vi "barebones control panel.vi"() -> ()   [LabVIEW 2012]
uses:
  JY-SPEX-TRIAX/controls.llb/Slits.ctl
  JY-SPEX-TRIAX/controls.llb/Turret Position (TRIAX).ctl
  Global/GPIB Numbers.vi
  JY-SPEX-TRIAX/JY-SPEX-TRIAX.lvlib
panel:
  out "wavelength at":dbl[unit]
  in  "Move to Wavelength":dbl[unit]
  in  "Read Wavelength":bool
  in  "Set Wavelength":bool
  in  "Read Grating":bool=TRUE
  out "Blaze Wavelength":dbl[unit]
  out "Groove Density":dbl[unit]
  in  "Set Grating":bool=TRUE
  in  "Grating position":T1
  in  "Set Mirror":bool=TRUE
  in  "position":enum16{"side (lateral)", "front (axial)"}(ring)
  in  "mirror":enum16{"entrance", "exit"}(ring)=enum."exit"
  in  "Read Slit":bool=TRUE
  out "Current Slit Position":dbl[unit]
  in  "Set Slit":bool=TRUE
  in  "Slit Entrance":T2
  in  "Desired Slit Position":dbl[unit]
  out "VISA out":refnum<visa-resource-name>
  out "error out":errorcluster
  in  "error in (no error)":errorcluster
  in  "Initialize":bool
  in  "stop":bool
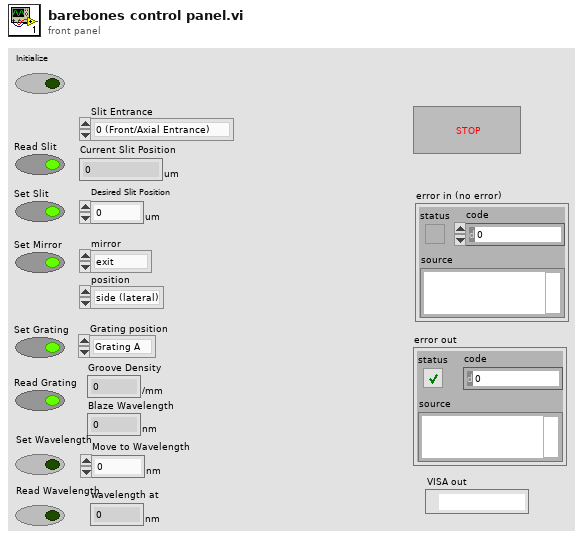
[diagram p1: front panel]
types:
  T1 = typedef "JY-SPEX-TRIAX.lvlib/Turret Position (TRIAX).ctl" = enum16{"Grating A", "Grating B", "Grating C"}
  T2 = typedef "JY-SPEX-TRIAX.lvlib/Slits.ctl" = enum16{"0 (Front/Axial Entrance)", "1 (Side/Lateral Entrance)", "2 (Front/Axial Exit)", "3 (Side/Lateral Exit)"}
  T3 = typedef "GPIB Type Def.ctl" = cluster{"Name":string, "bus":dbl, "GPIB":dbl, "GPIB as string":string, "byte":i32, "VISA Resource Name":refnum<visa-resource-name>}
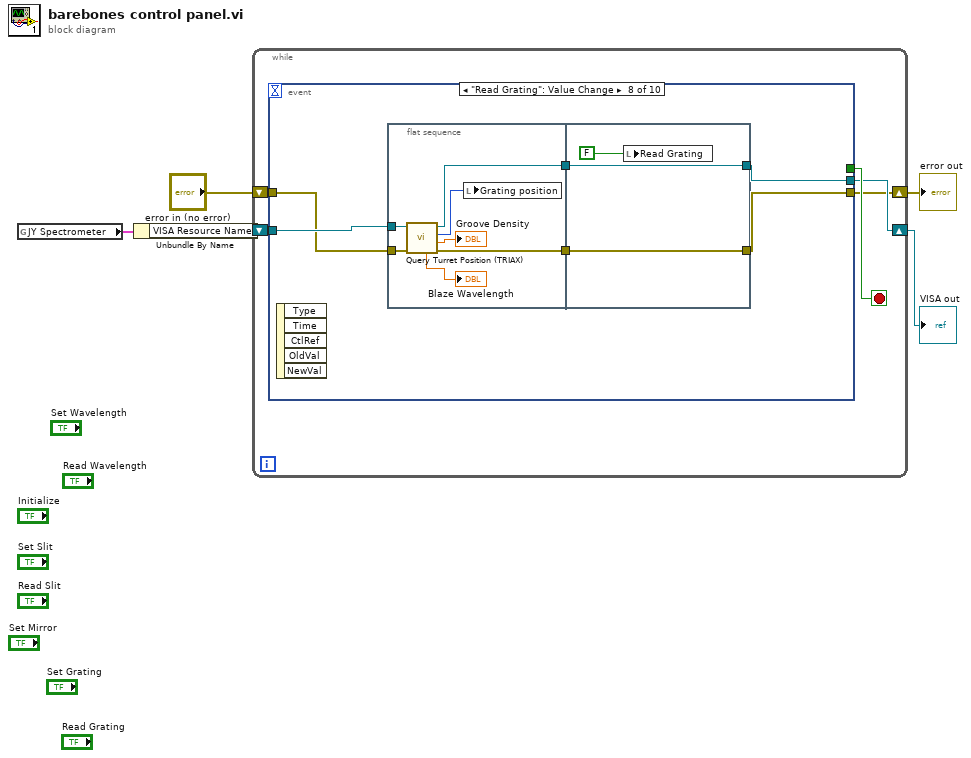
[diagram p0: block diagram]
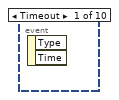
[diagram p2: hidden frame]
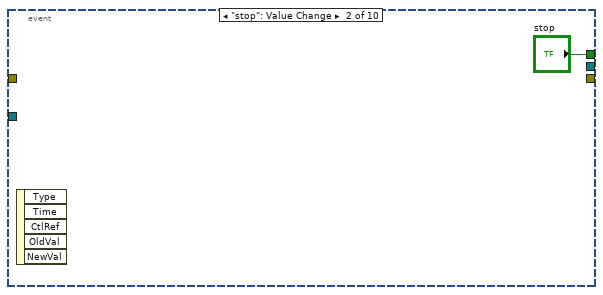
[diagram p3: hidden frame]
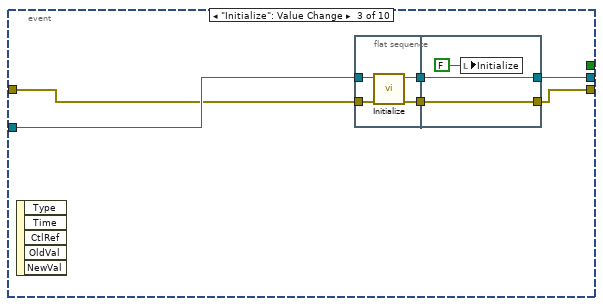
[diagram p4: hidden frame]
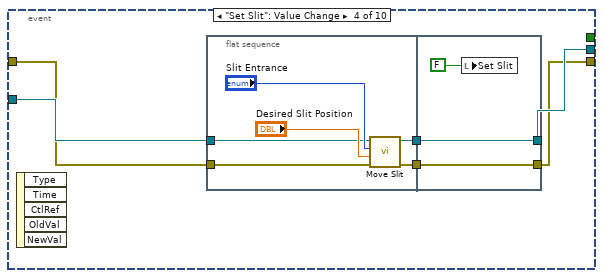
[diagram p5: hidden frame]
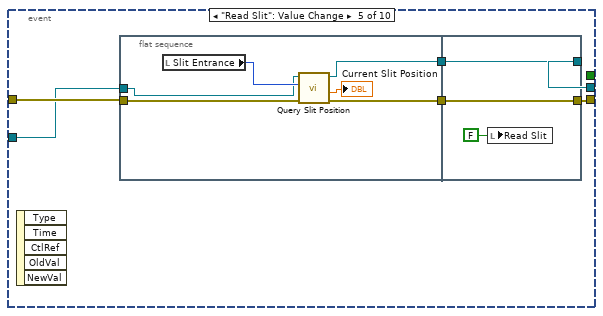
[diagram p6: hidden frame]
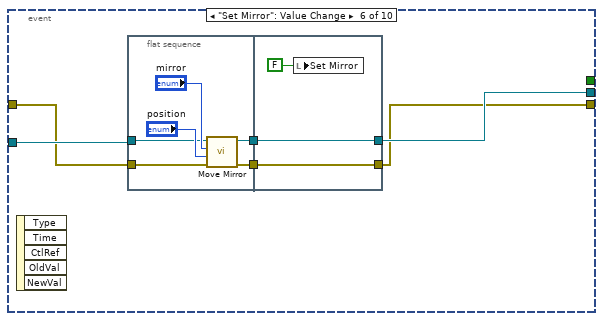
[diagram p7: hidden frame]
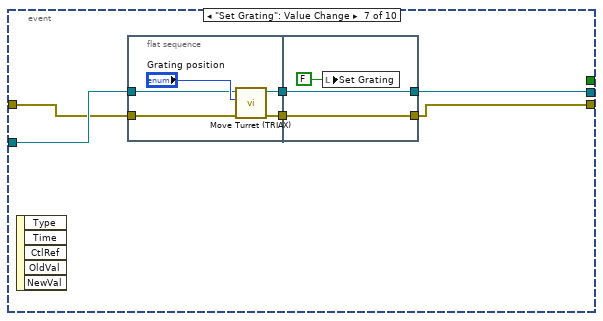
[diagram p8: hidden frame]
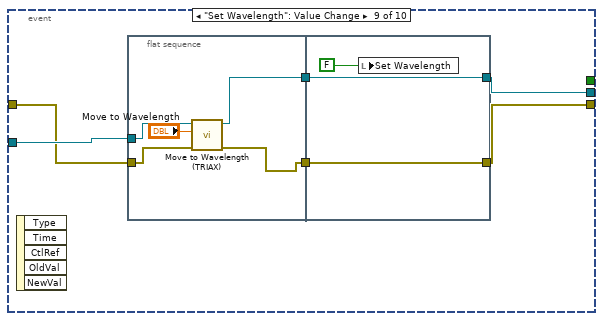
[diagram p9: hidden frame]
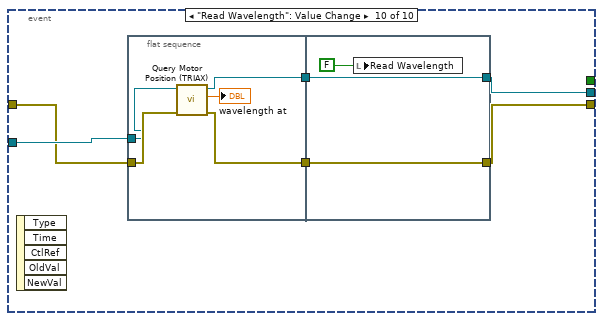
[diagram p10: hidden frame]
diagram:
  n1 = global read "GPIB Numbers.vi" "JY Spectrometer"() -> (w5:T3)
  n2 = Unbundle By Name(w5) -> ("VISA Resource Name"=w4:refnum<visa-resource-name>)
  n3 = while {
    shift-right: [w8] -> w1
    shift-left: w4 -> [w9]
    shift-right: [w6] -> w2
    shift-left: "error in (no error)" -> [w7]
    stop <- w10 stop-if-true
    n4 = event shown="[7] \"Read Grating\": Value Change" {
      selector: _ -> [_ _ _ _ _ _ _ _ _ _]
      dyn-events: _ -> [_ _ _ _ _ _ _ _ _ _]
      timeout: _ -> [_ _ _ _ _ _ _ _ _ _]
      tunnel: [_ "stop" _ _ _ _ _ _ _ _] -> w10
      tunnel: w9 -> [_ _ w17 w30 w42 w60 w75 w89 w105 w119]
      tunnel: w7 -> [_ _ w16 w27 w45 w59 w74 w88 w104 w118]
      tunnel: [_ _ w15 w29 w40 w57 w73 w87 w103 w117] -> w8
      tunnel: [_ _ w13 w26 w43 w55 w72 w86 w102 w116] -> w6
      event Timeout {
        n5 = event-data() -> ()  [unwired: 1 in, 2 out]
      }
      event "stop": Value Change {
        n6 = event-data() -> ()  [unwired: 1 in, 5 out]
      }
      event "Initialize": Value Change {
        n7 = event-data() -> ()  [unwired: 1 in, 5 out]
        n8 = flat-sequence {
          tunnel: w17 -> [w21]
          tunnel: w16 -> [w20]
          tunnel: [w19] -> w14
          tunnel: [w18] -> w12
          tunnel: [w23] -> w15
          tunnel: w14 -> [w23]
          tunnel: [w22] -> w13
          tunnel: w12 -> [w22]
          frame #0 {
            n9 = call "Initialize.vi"("error in (no error)"=w20, "VISA resource name"=w21) -> ("error out"=w18:errorcluster, "VISA resource name out"=w19:refnum<visa-resource-name>)  [unwired: 8 in]
          }
          frame #1 {
            n10 = local write "Initialize"(FALSE) -> ()
          }
        }
      }
      event "Set Slit": Value Change {
        n11 = event-data() -> ()  [unwired: 1 in, 5 out]
        n12 = flat-sequence {
          tunnel: w30 -> [w34]
          tunnel: [w33] -> w28
          tunnel: w27 -> [w32]
          tunnel: [w31] -> w25
          tunnel: [w38] -> w29
          tunnel: w28 -> [w38]
          tunnel: [w37] -> w26
          tunnel: w25 -> [w37]
          frame #0 {
            n13 = call "Move Slit.vi"("error in (no error)"=w32, "Desired Slit Position"="Desired Slit Position", "Slit (Front/Axial Entrance)"="Slit Entrance", "VISA resource name"=w34) -> ("error out"=w31:errorcluster, "VISA resource name out"=w33:refnum<visa-resource-name>)  [unwired: 6 in]
          }
          frame #1 {
            n14 = local write "Set Slit"(FALSE ("Move Slit")) -> ()
          }
        }
      }
      event "Read Slit": Value Change {
        n15 = event-data() -> ()  [unwired: 1 in, 5 out]
        n16 = flat-sequence {
          tunnel: w45 -> [w49]
          tunnel: [w48] -> w44
          tunnel: w42 -> [w47]
          tunnel: [w46] -> w41
          tunnel: [w54] -> w43
          tunnel: w44 -> [w54]
          tunnel: [w53] -> w40
          tunnel: w41 -> [w53]
          frame #0 {
            n17 = local read "Slit Entrance"() -> (w51:T2)
            n18 = call "Query Slit Position.vi"("error in (no error)"=w49, "Slit (Front/Axial Entrance)"=w51, "VISA resource name"=w47) -> ("error out"=w48:errorcluster, "Slit Position"=→"Current Slit Position":dbl[unit], "VISA resource name out"=w46:refnum<visa-resource-name>)  [unwired: 6 in]
          }
          frame #1 {
            n19 = local write "Read Slit"(FALSE ("Read Slit")) -> ()
          }
        }
      }
      event "Set Mirror": Value Change {
        n20 = event-data() -> ()  [unwired: 1 in, 5 out]
        n21 = flat-sequence {
          tunnel: w60 -> [w63]
          tunnel: w59 -> [w64]
          tunnel: [w62] -> w58
          tunnel: [w61] -> w56
          tunnel: [w68] -> w57
          tunnel: w58 -> [w68]
          tunnel: w56 -> [w67]
          tunnel: [w67] -> w55
          frame #0 {
            n22 = call "Move Mirror.vi"("error in (no error)"=w64, "position (side/lateral)"="position", "mirror (exit)"="mirror", "VISA resource name"=w63) -> ("error out"=w61:errorcluster, "VISA resource name out"=w62:refnum<visa-resource-name>)  [unwired: 6 in]
          }
          frame #1 {
            n23 = local write "Set Mirror"(FALSE ("Set Mirror 2")) -> ()
          }
        }
      }
      event "Set Grating": Value Change {
        n24 = event-data() -> ()  [unwired: 1 in, 5 out]
        n25 = flat-sequence {
          tunnel: w75 -> [w79]
          tunnel: w74 -> [w78]
          tunnel: [w77] -> w71
          tunnel: [w76] -> w70
          tunnel: [w83] -> w73
          tunnel: [w82] -> w72
          tunnel: w71 -> [w83]
          tunnel: w70 -> [w82]
          frame #0 {
            n26 = call "Move Turret (TRIAX).vi"("error in (no error)"=w78, "turret position (0)"="Grating position", "VISA resource name"=w79) -> ("error out"=w76:errorcluster, "VISA resource name out"=w77:refnum<visa-resource-name>)  [unwired: 7 in]
          }
          frame #1 {
            n27 = local write "Set Grating"(FALSE ("Set Grating")) -> ()
          }
        }
      }
      event "Read Grating": Value Change {
        n28 = event-data() -> ()  [unwired: 1 in, 5 out]
        n29 = flat-sequence {
          tunnel: w89 -> [w94]
          tunnel: w88 -> [w93]
          tunnel: [w92] -> w85
          tunnel: [w91] -> w84
          tunnel: [w99] -> w87
          tunnel: [w98] -> w86
          tunnel: w85 -> [w99]
          tunnel: w84 -> [w98]
          frame #0 {
            n30 = call "Query Turret Position (TRIAX).vi"("error in (no error)"=w93, "VISA resource name"=w94) -> ("error out"=w91:errorcluster, "Groove Density"=→"Groove Density":dbl[unit], "Turret Position"=w90:T1, "VISA resource name out"=w92:refnum<visa-resource-name>, "Blaze Wavelength"=→"Blaze Wavelength":dbl[unit])  [unwired: 5 in]
            n31 = local write "Grating position"(w90) -> ()
          }
          frame #1 {
            n32 = local write "Read Grating"(FALSE ("Set Grating")) -> ()
          }
        }
      }
      event "Set Wavelength": Value Change {
        n33 = event-data() -> ()  [unwired: 1 in, 5 out]
        n34 = flat-sequence {
          tunnel: w105 -> [w110]
          tunnel: w104 -> [w109]
          tunnel: [w107] -> w101
          tunnel: [w108] -> w100
          tunnel: [w113] -> w103
          tunnel: [w112] -> w102
          tunnel: w101 -> [w113]
          tunnel: w100 -> [w112]
          frame #0 {
            n35 = call "Move to Wavelength (TRIAX).vi"("error in (no error)"=w109, "Target wavelength"="Move to Wavelength", "VISA resource name"=w110) -> ("error out"=w108:errorcluster, "VISA resource name out"=w107:refnum<visa-resource-name>)  [unwired: 7 in]
          }
          frame #1 {
            n36 = local write "Set Wavelength"(FALSE ("Set Grating")) -> ()
          }
        }
      }
      event "Read Wavelength": Value Change {
        n37 = event-data() -> ()  [unwired: 1 in, 5 out]
        n38 = flat-sequence {
          tunnel: w119 -> [w121]
          tunnel: w118 -> [w122]
          tunnel: [w124] -> w115
          tunnel: [w123] -> w114
          tunnel: [w127] -> w117
          tunnel: [w126] -> w116
          tunnel: w115 -> [w127]
          tunnel: w114 -> [w126]
          frame #0 {
            n39 = call "Query Motor Position (TRIAX).vi"("error in (no error)"=w122, "VISA resource name"=w121) -> ("error out"=w123:errorcluster, "wavelength"=→"wavelength at":dbl[unit], "VISA resource name out"=w124:refnum<visa-resource-name>)  [unwired: 7 in]
          }
          frame #1 {
            n40 = local write "Read Wavelength"(FALSE ("Set Grating")) -> ()
          }
        }
      }
    }
  }
  "error out" <- w2
  "VISA out" <- w1
